vi "UnScaleValue.vi"(7 "physical channel":string, 8 "error in (no error)":errorcluster, 9 "Type&Value":cluster{"type":string, "Variant":variant}, 10 "Caps":T1, 11 "property":string) -> (0 "error out":errorcluster, 3 "Variant":variant)   [LabVIEW 2017]
uses:
  <vilib>/Utility/Data Type/NI_Data Type.lvlib
  API/Scale/Scale.lvlib
  Ctrl/TableScale.ctl
  Ctrl/Coercion.ctl
  Ctrl/PolynomialScale.ctl
  Ctrl/LinearScale.ctl
  API/Bitfield/Bitfield.lvlib
  API/Scale/Unscale(Linear).vi
  API/Scale/Unscale(Table).vi
  API/Scale/Unscale(Polynomial).vi
  Ctrl/Property.ctl
  Ctrl/PhysicalChannel.ctl
  Ctrl/Bitfield.ctl
  Ctrl/Register.ctl
  Ctrl/ScaleType.ctl
  Ctrl/Scale.ctl
  Ctrl/EnumValue.ctl
  Ctrl/Enum.ctl
  Ctrl/Caps.ctl
panel:
  out "dataType":string
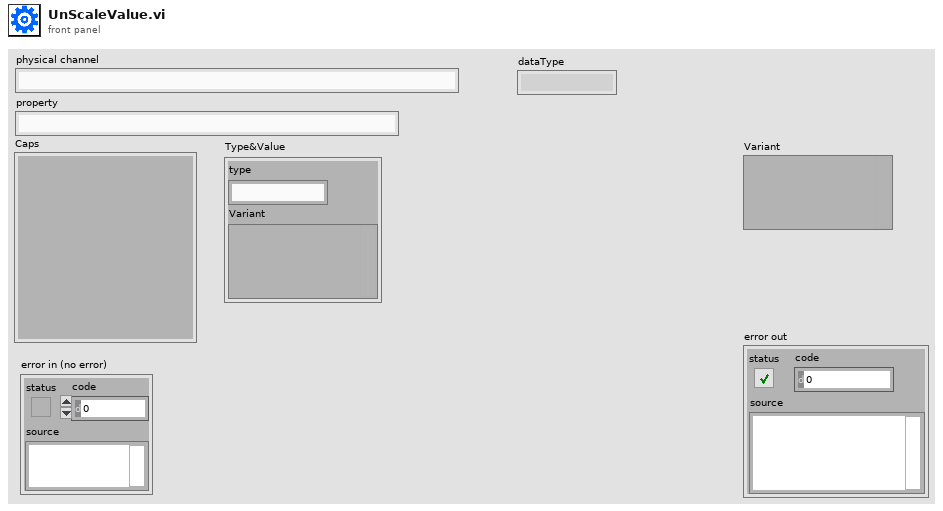
[diagram p1: front panel]
types:
  T1 = typedef "Caps.ctl" = cluster{"properties":T2[], "physical channels":T3[], "registers":T4[], "scales":T6[], "enums":T8[], "productName":string}
  T2 = typedef "Property.ctl" = cluster{"name":string, "bitfield":string, "value":variant, "dataType":string, "min":variant, "max":variant, "scale":string, "access":string}
  T3 = typedef "PhysicalChannel.ctl" = cluster{"name":string, "properties":T2[]}
  T4 = typedef "Register.ctl" = cluster{"name":string, "address":i32, "size":i32, "bitfields":T5[], "initialValue":variant, "connectedProperties":string[]}
  T5 = typedef "Bitfield.ctl" = cluster{"name":string, "offset":i32, "size":i32, "signed":bool}
  T6 = typedef "Scale.ctl" = cluster{"name":string, "type":T7, "params":variant}
  T7 = typedef "ScaleType.ctl" = enum16{"NoScale", "Table", "Polynomial", "Linear"}
  T8 = typedef "Enum.ctl" = cluster{"name":string, "values":T9[]}
  T9 = typedef "EnumValue.ctl" = cluster{"name":string, "value":i32}
  T10 = cluster{"Property":T2, "register":T4, "bitfield":T5, "scale":T6, "enum":T8}
  T11 = typedef "TableScale.ctl" = cluster{"name":string, "coercion":string, "table":cluster{"scaled":dbl, "unscaled":dbl}[]}
  T12 = typedef "Coercion.ctl" = enum16{"Strict", "RoundToNearest", "Interpolate"}
  T13 = typedef "PolynomialScale.ctl" = cluster{"name":string, "forwardCoeffs":dbl[], "reverseCoeffs":dbl[]}
  T14 = typedef "LinearScale.ctl" = cluster{"name":string, "m":dbl, "b":dbl}
  T15 = typedef "NI_Data Type.lvlib/Data Type.ctl" = enum8{"Invalid Type", "Void", "I8", "I16", "I32", "I64", "U8", "U16", "U32", "U64", "Single Float", "Double Float", "Extended Float", "Single Complex", "Double Complex", "Extended Complex", "Enum U8", "Enum U16", "Enum U32", "Enum U64", "Single Float With Unit", "Double Float With Unit", "Extended Float With Unit", "Single Complex with Unit", "Double Complex with Unit", "Extended Complex with Unit", "Boolean", "String", "Path", "Picture", "Tag", "Array", "Cluster", "Variant", "LV Variant", "Waveform", "Timestamp", "Digital Waveform", "Digital Data", "ExpressData", "Refnum", "External Data", "VI", "Poly VI", "LabVIEW Class Instance", "Fixed Point"}
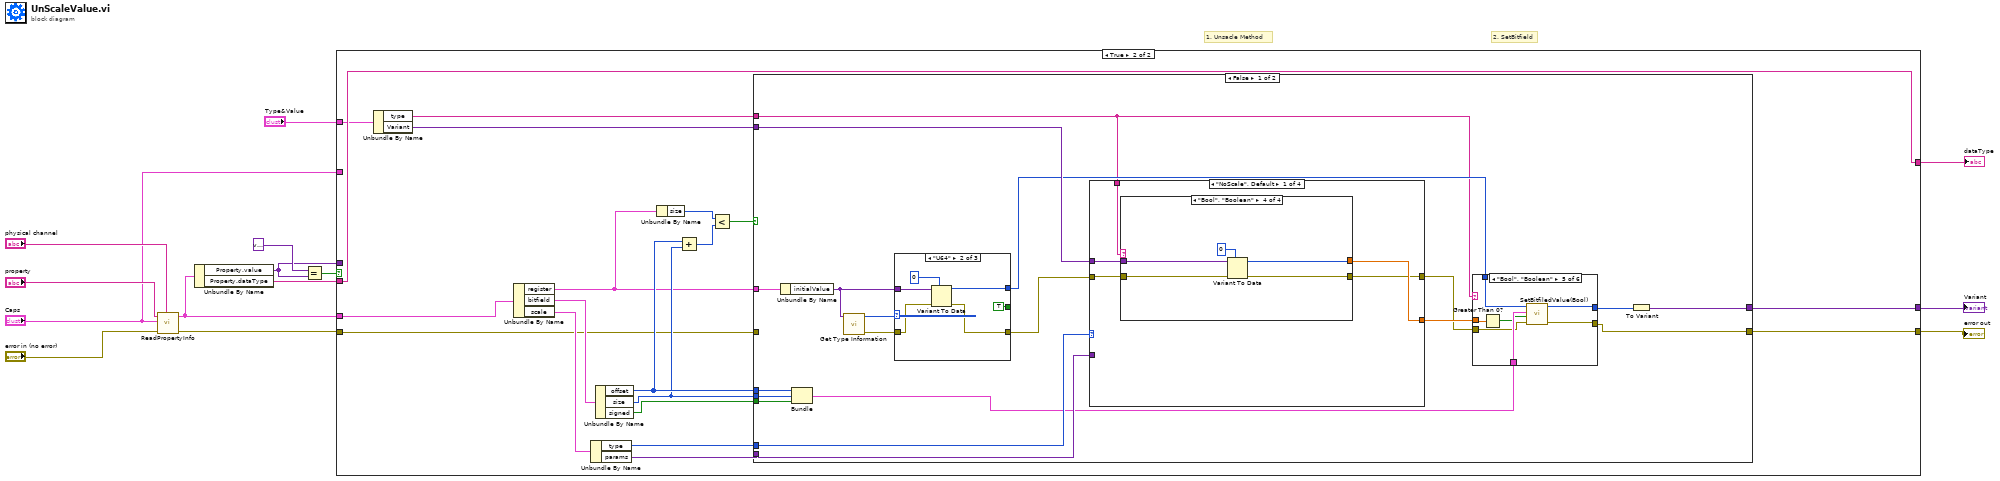
[diagram p0: block diagram]
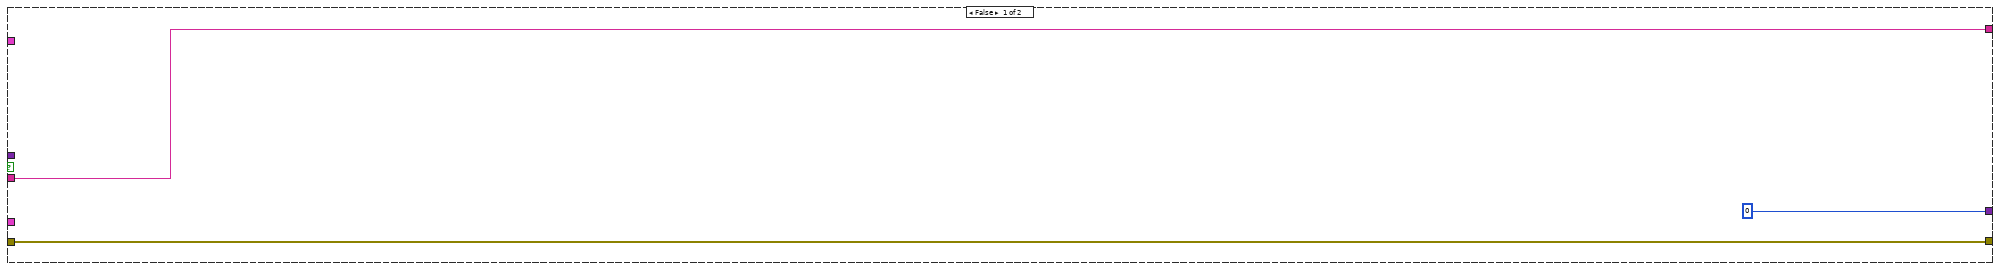
[diagram p2: hidden frame]
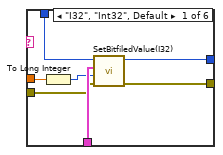
[diagram p3: hidden frame]
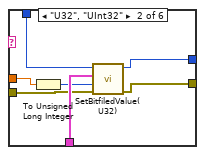
[diagram p4: hidden frame]
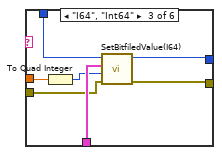
[diagram p5: hidden frame]
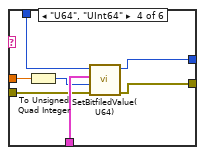
[diagram p6: hidden frame]
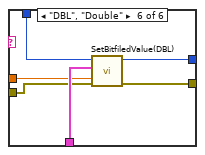
[diagram p7: hidden frame]
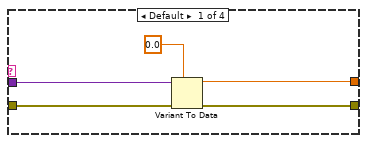
[diagram p8: hidden frame]
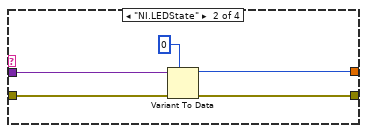
[diagram p9: hidden frame]
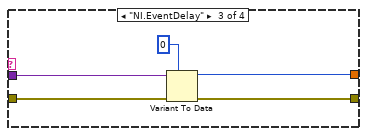
[diagram p10: hidden frame]
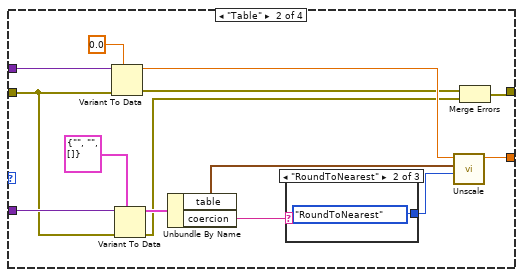
[diagram p11: hidden frame]
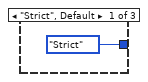
[diagram p12: hidden frame]
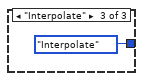
[diagram p13: hidden frame]
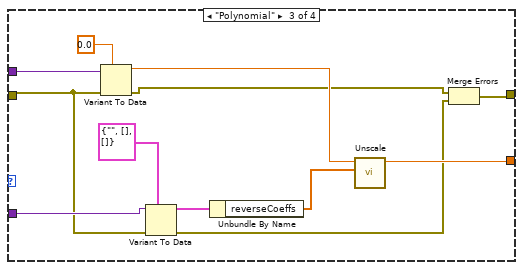
[diagram p14: hidden frame]
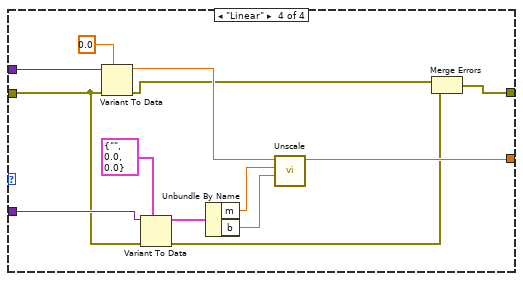
[diagram p15: hidden frame]
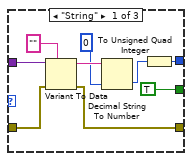
[diagram p16: hidden frame]
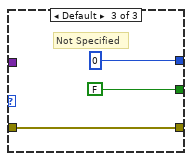
[diagram p17: hidden frame]
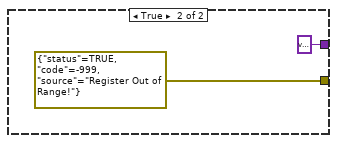
[diagram p18: hidden frame]
diagram:
  # "2. SetBitfield"
  # "1. Unsacle Method"
  n1 = call "ReadPropertyInfo.vi"("physical channel"="physical channel", "error in (no error)"="error in (no error)", "Caps"="Caps", "property"="property") -> ("error out"=w12:errorcluster, "property info"=w11:T10)  [unwired: 6 in]
  n2 = Unbundle By Name(w11) -> ("Property.value"=w7:variant, "Property.dataType"=w8:string)
  n3 = Equal?(x=variant, y=w7) -> (x = y?=w9:bool)
  n4 = case shown="True" w9 {
    tunnel: w11 -> [_ w28]
    tunnel: [w17 w25] -> w13
    tunnel: [w16 w33] -> w4
    tunnel: w12 -> [w17 w18]
    tunnel: w8 -> [w16 w33]
    tunnel: w7 -> [_ _]
    tunnel: "Type&Value" -> [_ w32]
    tunnel: "Caps" -> [_ _]
    tunnel: [u64 0 ("update value") w27] -> w1
    frame False {
    }
    frame True {
      n5 = Unbundle By Name(w32) -> ("type"=w26:string, "Variant"=w29:variant)
      n6 = Unbundle By Name(w28) -> ("register"=w22:T4, "bitfield"=w36:T5, "scale"=w35:T6)
      n7 = Unbundle By Name(w35) -> ("type"=w31:T7, "params"=w30:variant)
      n8 = Unbundle By Name(w36) -> ("offset"=w24:i32, "size"=w23:i32, "signed"=w34:bool)
      n9 = Unbundle By Name(w22) -> ("size"=w21:i32)
      n10 = Add(x=w24, y=w23) -> (x+y=w20:i32)
      n11 = Less?(x=w21, y=w20) -> (x < y?=w19:bool)
      n12 = case shown="False" w19 {
        tunnel: w24 -> [w55 _]
        tunnel: w34 -> [w54 _]
        tunnel: w23 -> [w53 _]
        tunnel: w22 -> [w52 _]
        tunnel: w31 -> [w48 _]
        tunnel: w30 -> [w47 _]
        tunnel: w29 -> [w46 _]
        tunnel: [w39 variant ("Variant")] -> w27
        tunnel: w26 -> [w38 _]
        tunnel: [w37 errorcluster {"status"=TRUE, "code"=-999, "source"="Register Out of Range!"} ("error out")] -> w25
        tunnel: w18 -> [_ _]
        frame False {
          n13 = Unbundle By Name(w52) -> ("initialValue"=w49:variant)
          n14 = Bundle("offset"=w55, "size"=w53, "signed"=w54) -> (w45:cluster{"offset":i32, "size":i32, "signed":bool})  [unwired: 1 in]
          n15 = call <vilib>:"Get Type Information.vi"("Variant"=w49) -> ("error out"=w50:errorcluster, "Type"=w51:T15)  [unwired: 6 in, 3 out]
          n16 = case shown="\"U64\"" w51 {
            tunnel: [w170 w177 u64 0] -> w44
            tunnel: w49 -> [w167 w175 _]
            tunnel: w50 -> [w166 w176 w180]
            tunnel: [w165 w173 w180] -> w41
            tunnel: [TRUE TRUE FALSE] -> _
            frame "String" {
              n17 = Variant To Data(error in=w166, type="", Variant=w167) -> (data=w171:string, error out=w165:errorcluster)
              n18 = Decimal String To Number(string=w171, default (0L)=u64 0 ("default (0 I32)")) -> (number=w169:u64)  [unwired: 1 in, 1 out]
              n19 = To Unsigned Quad Integer(1:w169) -> (0:w170:u64)
            }
            frame "U64" {
              n20 = Variant To Data(error in=w176, type=u64 0, Variant=w175) -> (data=w177:u64, error out=w173:errorcluster)
            }
            frame Default {
              # "Not Specified"
            }
          }
          n21 = case shown="\"NoScale\", Default" w48 {
            tunnel: w47 -> [_ w134 w148 w159]
            tunnel: w46 -> [w101 w129 w144 w162]
            tunnel: [w100 w126 w150 w155] -> w43
            tunnel: w41 -> [w99 w125 w142 w154]
            tunnel: [w98 w124 w141 w153] -> w40
            tunnel: w38 -> [w97 _ _ _]
            frame "NoScale", Default {
              n22 = case shown="\"Bool\", \"Boolean\"" w97 {
                tunnel: w101 -> [w106 w110 w115 w117]
                tunnel: [w104 w108 w113 w119] -> w100
                tunnel: w99 -> [w103 w109 w114 w121]
                tunnel: [w102 w107 w112 w118] -> w98
                frame Default {
                  n23 = Variant To Data(error in=w103, type=0.0, Variant=w106) -> (data=w104:dbl, error out=w102:errorcluster)
                }
                frame "NI.LEDState" {
                  n24 = Variant To Data(error in=w109, type=0 ("Value"), Variant=w110) -> (data=w108:i32, error out=w107:errorcluster)
                }
                frame "NI.EventDelay" {
                  n25 = Variant To Data(error in=w114, type=0 ("Value"), Variant=w115) -> (data=w113:i32, error out=w112:errorcluster)
                }
                frame "Bool", "Boolean" {
                  n26 = Variant To Data(error in=w121, type=u16 0, Variant=w117) -> (data=w119:u16, error out=w118:errorcluster)
                }
              }
            }
            frame "Table" {
              n27 = Variant To Data(error in=w125, type=0.0, Variant=w129) -> (data=w127:dbl, error out=w123:errorcluster)
              n28 = Variant To Data(error in=w125, type=T11 {"name"="", "coercion"="", "table"=[]} ("TableScale"), Variant=w134) -> (data=w133:T11, error out=w122:errorcluster)
              n29 = Unbundle By Name(w133) -> ("table"=w131:cluster{"scaled":dbl, "unscaled":dbl}[], "coercion"=w132:string)
              n30 = case shown="\"RoundToNearest\"" w132 {
                tunnel: [Coercion."Strict" ("coercion") Coercion."RoundToNearest" ("coercion") Coercion."Interpolate" ("coercion")] -> w130
                frame "Strict", Default {
                }
                frame "RoundToNearest" {
                }
                frame "Interpolate" {
                }
              }
              n31 = call-poly "Unscale.vi"("coercion"=w130, "scales"=w131, "scale value"=w127) -> ("unscale value"=w126:dbl)  [unwired: 8 in]
              n32 = Merge Errors(w123, w122) -> (w124:errorcluster)
            }
            frame "Polynomial" {
              n33 = Variant To Data(error in=w142, type=0.0, Variant=w144) -> (data=w143:dbl, error out=w140:errorcluster)
              n34 = Variant To Data(error in=w142, type=T13 {"name"="", "forwardCoeffs"=[], "reverseCoeffs"=[]} ("PolynomialScale"), Variant=w148) -> (data=w147:T13, error out=w139:errorcluster)
              n35 = Unbundle By Name(w147) -> ("reverseCoeffs"=w146:dbl[])
              n36 = call-poly "Unscale.vi"("reverse coeffs"=w146, "scaled value"=w143) -> ("unscaled value"=w150:dbl)  [unwired: 9 in]
              n37 = Merge Errors(w140, w139) -> (w141:errorcluster)
            }
            frame "Linear" {
              n38 = Variant To Data(error in=w154, type=0.0, Variant=w162) -> (data=w161:dbl, error out=w152:errorcluster)
              n39 = Variant To Data(error in=w154, type=T14 {"name"="", "m"=0.0, "b"=0.0} ("LinearScale"), Variant=w159) -> (data=w158:T14, error out=w151:errorcluster)
              n40 = Unbundle By Name(w158) -> ("m"=w157:dbl, "b"=w156:dbl)
              n41 = call-poly "Unscale.vi"("offset"=w156, "multiplier"=w157, "scaled value"=w161) -> ("unscaled value"=w155:dbl)  [unwired: 8 in]
              n42 = Merge Errors(w152, w151) -> (w153:errorcluster)
            }
          }
          n43 = case shown="\"Bool\", \"Boolean\"" w38 {
            tunnel: w45 -> [w62 w68 w76 w81 w89 w95]
            tunnel: w44 -> [w61 w69 w75 w82 w90 w96]
            tunnel: w43 -> [w60 w67 w74 w83 w88 w94]
            tunnel: [w58 w65 w72 w79 w86 w93] -> w42
            tunnel: w40 -> [w57 w64 w71 w78 w85 w92]
            tunnel: [w56 w63 w70 w77 w84 w91] -> w37
            frame "I32", "Int32", Default {
              n44 = To Long Integer(number=w60) -> (32bit integer=w59:i32)
              n45 = call "SetBitfiledValue(I32).vi"("error in (no error)"=w57, "bitfield value"=w59, "bitfield caps"=w62, "original value"=w61) -> ("error out"=w56:errorcluster, "update value"=w58:u64)  [unwired: 6 in]
            }
            frame "U32", "UInt32" {
              n46 = To Unsigned Long Integer(number=w67) -> (unsigned 32bit integer=w66:u32)
              n47 = call "SetBitfiledValue(U32).vi"("error in (no error)"=w64, "bitfield value"=w66, "bitfield caps"=w68, "original value"=w69) -> ("error out"=w63:errorcluster, "update value"=w65:u64)  [unwired: 6 in]
            }
            frame "I64", "Int64" {
              n48 = To Quad Integer(1:w74) -> (0:w73:i64)
              n49 = call "SetBitfiledValue(I64).vi"("error in (no error)"=w71, "bitfield value"=w73, "bitfield caps"=w76, "original value"=w75) -> ("error out"=w70:errorcluster, "update value"=w72:u64)  [unwired: 6 in]
            }
            frame "U64", "UInt64" {
              n50 = To Unsigned Quad Integer(1:w83) -> (0:w80:u64)
              n51 = call "SetBitfiledValue(U64).vi"("error in (no error)"=w78, "bitfield value"=w80, "bitfield caps"=w81, "original value"=w82) -> ("error out"=w77:errorcluster, "update value"=w79:u64)  [unwired: 6 in]
            }
            frame "Bool", "Boolean" {
              n52 = Greater Than 0?(x=w88) -> (x > 0?=w87:bool)
              n53 = call "SetBitfiledValue(Bool).vi"("error in (no error)"=w85, "bitfield value"=w87, "bitfield caps"=w89, "original value"=w90) -> ("error out"=w84:errorcluster, "update value"=w86:u64)  [unwired: 6 in]
            }
            frame "DBL", "Double" {
              n54 = call "SetBitfiledValue(DBL).vi"("error in (no error)"=w92, "bitfield value"=w94, "bitfield caps"=w95, "original value"=w96) -> ("error out"=w91:errorcluster, "update value"=w93:u64)  [unwired: 6 in]
            }
          }
          n55 = To Variant(anything=w42) -> (Variant=w39:variant)
        }
        frame True {
        }
      }
    }
  }
  "error out" <- w13
  "dataType" <- w4
  "Variant" <- w1
